vi "SendRS232Command.vi"(8 "error in (no error)":errorcluster, 10 "Command":string, 11 "VISA/RS232 Device In":refnum<visa-resource-name>) -> (0 "error out":errorcluster, 3 "VISA/RS232 Device Out":refnum<visa-resource-name>)   [LabVIEW 2017]
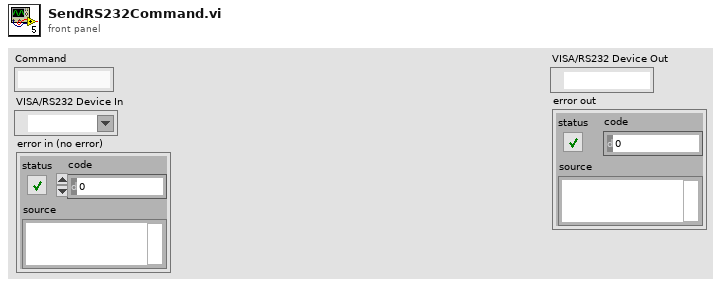
[diagram p1: front panel]
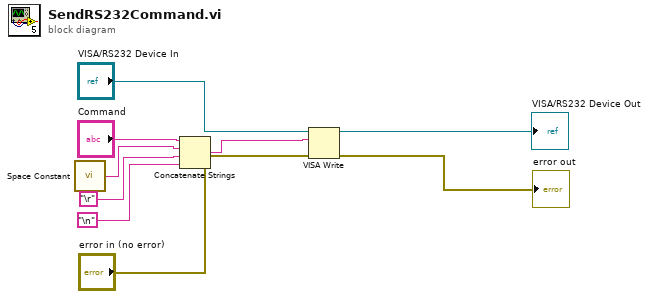
[diagram p0: block diagram]
diagram:
  n1 = call <vilib>:"Space Constant.vi"() -> ("String"=w7:string)
  n2 = Concatenate Strings("Command", w7, "\r", "\n") -> (w4:string)
  n3 = VISA Write(VISA resource name="VISA/RS232 Device In", write buffer=w4, error in (no error)="error in (no error)") -> (VISA resource name out=→"VISA/RS232 Device Out":refnum<visa-resource-name>, error out=→"error out":errorcluster)  [unwired: 1 out]
